vi "System Exec+.vi"(8 "error in (no error)":errorcluster, 9 "wait until closed? (F)":bool, 10 "run minimized? (F)":bool, 11 "command line to execute (\"\")":string) -> (0 "error out":errorcluster)   [LabVIEW 2023, in "Winevent.lvlib"]
doc: "This VI will launch another application as if you used the Run... command from Program Manager's or File Manager's File menu. If the wait until closed? setting is TRUE, the VI will wait until you close the application before continuing.\n\nYou can also choose how the window for the application will appear (for Windows applications only) with the run minimized? input.\n\nIf an error occurs, the code is returned in the error cluster."
uses:
  Winevent.lvlib
  LVWUtil32.dll
panel:
  in  "timeout (ms) (60000)":i32=60000
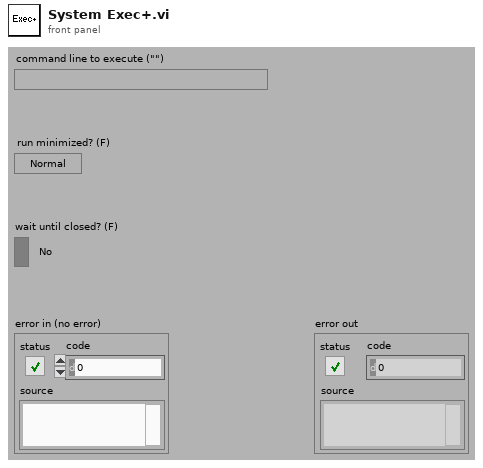
[diagram p1: front panel]
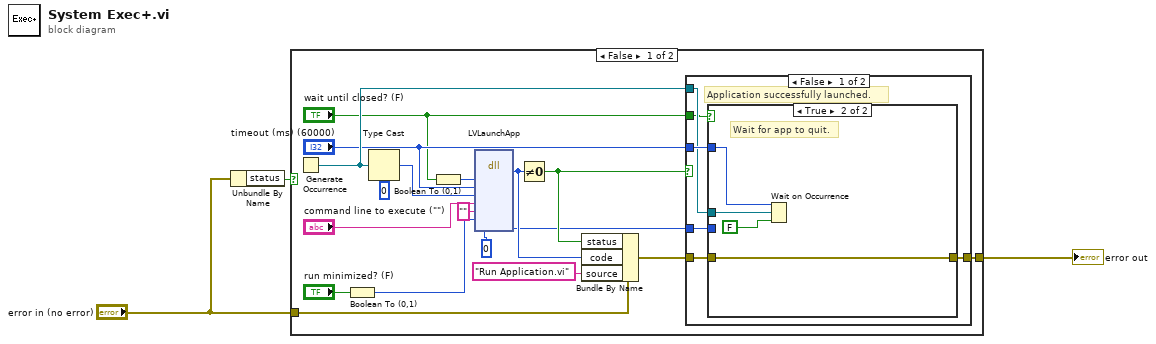
[diagram p0: block diagram]
diagram:
  n1 = Unbundle By Name("error in (no error)") -> ("status"=w3:bool)
  n2 = case shown="False" w3 {
    tunnel: "error in (no error)" -> [w20 w36]
    tunnel: [w17 w36] -> w2
    frame False {
      n3 = Generate Occurrence() -> (w8:refnum<k4>)
      n4 = Boolean To (0,1)(Boolean="run minimized? (F)") -> (0, 1=w10:i16)
      n5 = Type Cast(type=0, x=w8) -> (*(type *) &x=w12:i32)
      n6 = Boolean To (0,1)(Boolean="wait until closed? (F)") -> (0, 1=w14:i16)
      n7 = dll-call lib="C:/Users/acasalen/Documents/LabVIEW Data/Projects/Reds-Auto-Clicker/Red's Auto Clicker/SubVIs/labview_win_util32_8.6/LVWUtil32.dll" fn="LVLaunchApp"("bWait"=w14, "lTimeout"="timeout (ms) (60000)", "oRefNum"=w12, "lpszCommandLine"="command line to execute (\"\")", "lpszWorkDir"="", "bRunMinimized"=w10, "processId"=u32 0) -> (w15:i32, "processId"=w5:u32)  [unwired: 8 in, 3 out]
      n8 = Not Equal To 0?(x=w15) -> (x != 0?=w16:bool)
      n9 = Bundle By Name(cluster=w20, "status"=w16, "code"=w15, "source"="Run Application.vi") -> (w18:errorcluster)
      n10 = case shown="False" w16 {
        tunnel: w18 -> [w27 w33]
        tunnel: [w26 w33] -> w17
        tunnel: w8 -> [w24 _]
        tunnel: "timeout (ms) (60000)" -> [w25 _]
        tunnel: "wait until closed? (F)" -> [w23 _]
        tunnel: w5 -> [w22 _]
        frame False {
          # "Application successfully launched."
          n11 = case shown="True" w23 {
            tunnel: w27 -> [w28 w32]
            tunnel: [w28 w32] -> w26
            tunnel: w25 -> [_ w29]
            tunnel: w24 -> [_ w30]
            tunnel: w22 -> [_ _]
            frame False {
            }
            frame True {
              # "Wait for app to quit."
              n12 = Wait on Occurrence(1:FALSE, 2:w30, 3:w29) -> ()  [unwired: 1 out]
            }
          }
        }
        frame True {
          # "Error"
        }
      }
    }
    frame True {
      # "Error in.  Do nothing."
      n13 = Initialize Array("", 0) -> ()  [unwired: 1 out]
    }
  }
  "error out" <- w2
